vi "Configure AC Sample Method.vi"(8 "error in (no error)":errorcluster, 9 "Enable Ratio Measurement(Enable)":bool=TRUE, 10 "AC Sample Method (0: Analog)":u16(ring) items=["Analog", "Random", "Synchronous"], 11 "VISA resource name":refnum<visa-resource-name>) -> (0 "error out":errorcluster, 3 "VISA resource name out":refnum<visa-resource-name>)   [LabVIEW 2020, in "Agilent 3458.lvlib"]
doc: "Configures how the DMM makes true RMS AC voltage or AC + DC voltage measurements. The three options(synchronous, analog and random) all have different frequency ranges, best accuracy values and different readings per second values. Consult the manual to choose which option is best suited for your measurements."
uses:
  Agilent 3458.lvlib
panel:
  # "YES"
  # "NO"
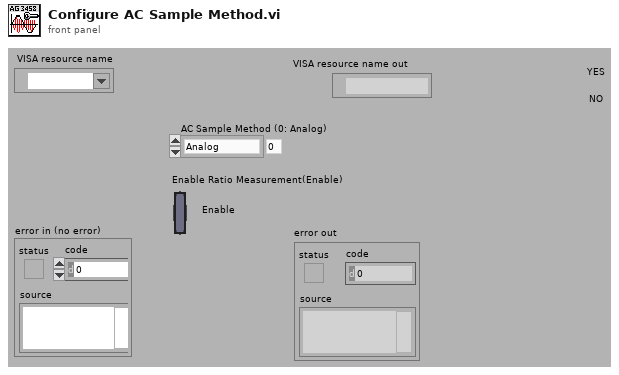
[diagram p1: front panel]
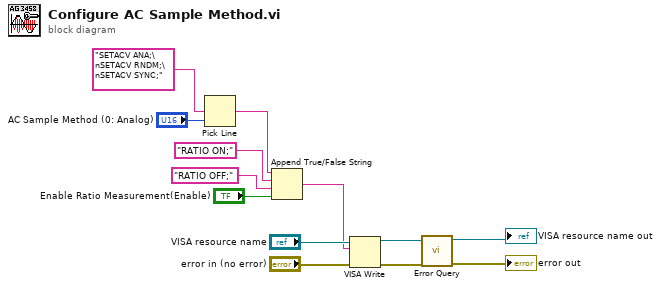
[diagram p0: block diagram]
diagram:
  n1 = Pick Line(multi-line string="SETACV ANA;\nSETACV RNDM;\nSETACV SYNC;", line index="AC Sample Method (0: Analog)") -> (output string=w4:string)  [unwired: 1 in]
  n2 = Append True/False String(1:"Enable Ratio Measurement(Enable)", 2:"RATIO OFF;", 3:"RATIO ON;", 4:w4) -> (0:w3:string)
  n3 = VISA Write(VISA resource name="VISA resource name", write buffer=w3, error in (no error)="error in (no error)") -> (VISA resource name out=w12:refnum<visa-resource-name>, error out=w11:errorcluster)  [unwired: 1 out]
  n4 = call "Error Query.vi"("error in (no error)"=w11, "VISA resource name"=w12) -> ("error out"=→"error out":errorcluster, "VISA resource name out"=→"VISA resource name out":refnum<visa-resource-name>)  [unwired: 6 in, 2 out]
